vi "Control Simu.vi"(6 "Error Feedback":bool, 7 "Watchdog Feedback In":i32, 10 "Error Ch":bool[](array[boolean]), 11 "Controls In":T2) -> (3 "Controls Out":T1, 4 "Error Feedback out":bool, 5 "Watchdog Feedback Out":i32)   [LabVIEW 2026]
uses:
  C:/Program Files/National Instruments/AMS plugin/Capabilities/Capabilities/High Level Capabilities/Power Supply Cluster/Producer Control.ctl
  C:/Program Files/National Instruments/AMS plugin/Capabilities/Capabilities/High Level Capabilities/Power Supply Cluster/Power Supply Cluster.lvclass
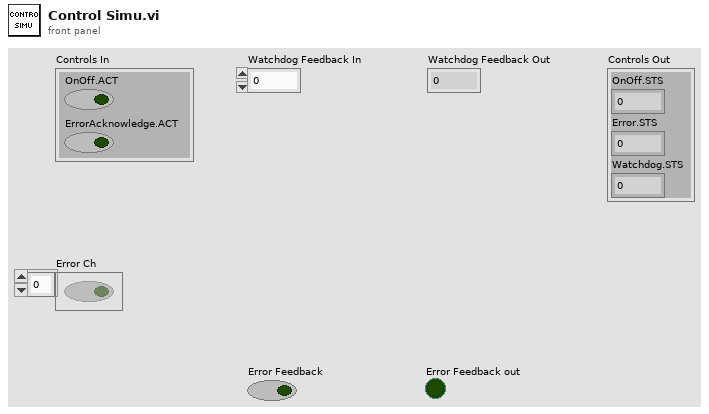
[diagram p1: front panel]
types:
  T1 = typedef "Power Supply Cluster.lvclass/Producer Control.ctl" = cluster{"OnOff.STS":i32, "Error.STS":i32, "Watchdog.STS":i32}
  T2 = cluster{"OnOff.ACT":bool, "ErrorAcknowledge.ACT":bool}
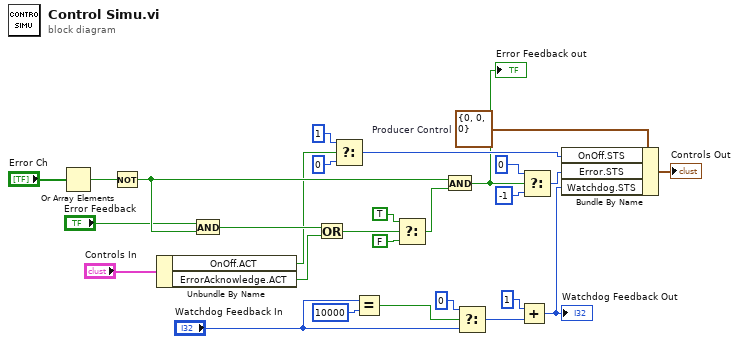
[diagram p0: block diagram]
diagram:
  w2 = T1 {"OnOff.STS"=0, "Error.STS"=0, "Watchdog.STS"=0}  # Producer Control
  n1 = Or Array Elements(Boolean array="Error Ch") -> (logical OR=w22:bool)
  n2 = Not(x=w22) -> (.not. x?=w25:bool)
  n3 = Unbundle By Name("Controls In") -> ("OnOff.ACT"=w11:bool, "ErrorAcknowledge.ACT"=w10:bool)
  n4 = And(x="Error Feedback", y=w25) -> (x .and. y?=w26:bool)
  n5 = Or(x=w26, y=w10) -> (x .or. y?=w23:bool)
  n6 = Select(t=1, s=w11, f=0) -> (s? t:f=w8:i32)
  n7 = Equal?(x="Watchdog Feedback In", y=10000) -> (x = y?=w27:bool)
  n8 = Select(t=TRUE, s=w23, f=FALSE) -> (s? t:f=w24:bool)
  n9 = And(x=w25, y=w24) -> (x .and. y?=w4:bool)
  "Error Feedback out" <- w4
  n10 = Select(t=0, s=w27, f="Watchdog Feedback In") -> (s? t:f=w28:i32)
  n11 = Add(x=1, y=w28) -> (x+y=w5:i32)
  "Watchdog Feedback Out" <- w5
  n12 = Select(t=0, s=w4, f=-1) -> (s? t:f=w9:i32)
  n13 = Bundle By Name(cluster=w2, "OnOff.STS"=w8, "Error.STS"=w9, "Watchdog.STS"=w5) -> (→"Controls Out":T1)
